vi "SUB_SFCSIPEI_convert.vi"(3 "SFCS IPEI String":string="04076 0097188 *") -> (1 "OutputString":string)   [LabVIEW 2011]
panel:
  # "因為DUT IPEI 如果尾數是10 ,在系統是用* 表示"
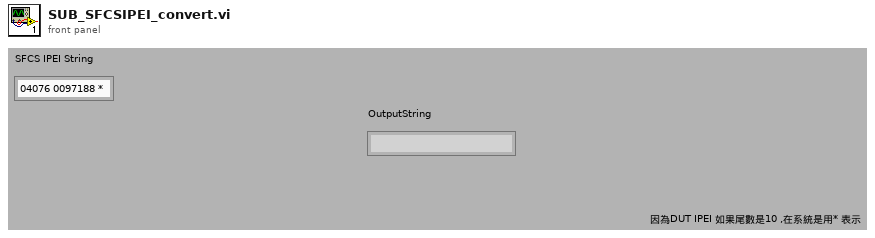
[diagram p1: front panel]
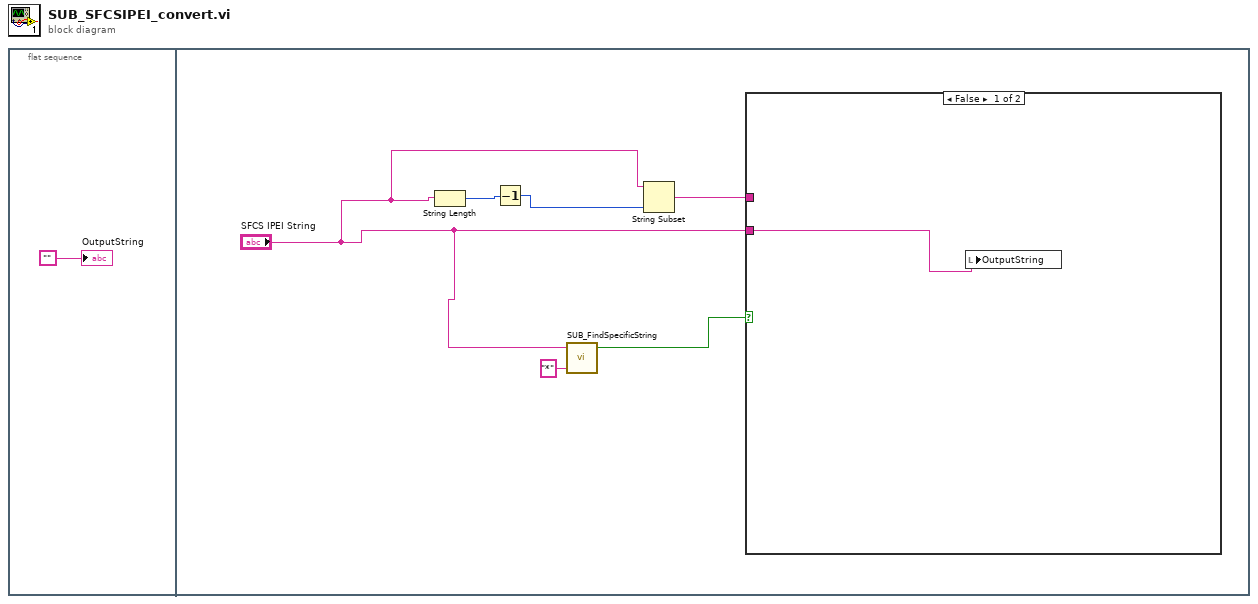
[diagram p0: block diagram]
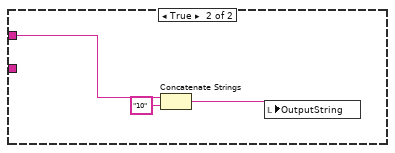
[diagram p2: hidden frame]
diagram:
  n1 = flat-sequence {
    frame #0 {
      "OutputString" <- ""
    }
    frame #1 {
      n2 = String Length(string="SFCS IPEI String") -> (length=w5:i32)
      n3 = Decrement(x=w5) -> (x-1=w4:i32)
      n4 = call "SUB_FindSpecificString.vi"("Find this String"="*", "String data"="SFCS IPEI String") -> ("Found"=w6:bool)  [unwired: 2 in, 1 out]
      n5 = String Subset(string="SFCS IPEI String", length (rest)=w4) -> (substring=w3:string)  [unwired: 1 in]
      n6 = case shown="False" w6 {
        tunnel: w3 -> [_ w11]
        tunnel: "SFCS IPEI String" -> [w8 _]
        frame False {
          n7 = local write "OutputString"(w8) -> ()
        }
        frame True {
          n8 = Concatenate Strings(w11, "10" ("string")) -> (w9:string)
          n9 = local write "OutputString"(w9) -> ()
        }
      }
    }
  }
